vi "Plot Closed.vi"(8 "error in (no error)":errorcluster, 10 "Closed plot":refnum<class "Message Enqueuer.lvclass">, 11 "Measure Controller in":refnum<class "Measure Controller.lvclass">) -> (0 "error out":errorcluster, 3 "Measure Controller out":refnum<class "Measure Controller.lvclass">)   [LabVIEW 2015, in "Measure Controller.lvclass"]
uses:
  Measure Controller.lvclass
  <vilib>/ActorFramework/Message Enqueuer/Message Enqueuer.lvclass
  Measure Controller.lvclass/Measure Controller.ctl
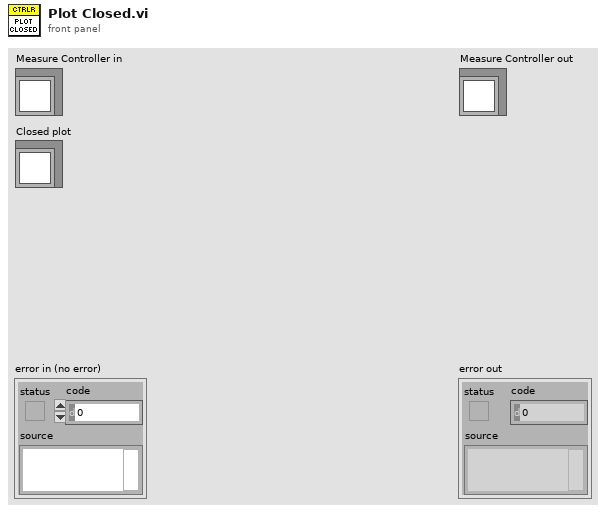
[diagram p1: front panel]
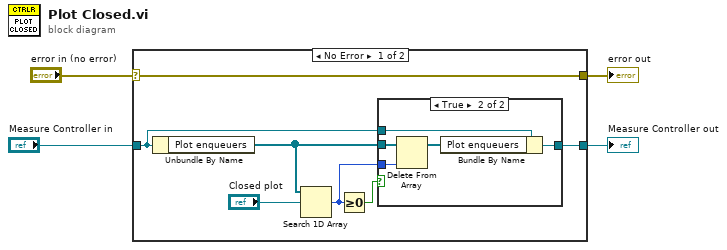
[diagram p0: block diagram]
diagram:
  n1 = case shown="No Error" "error in (no error)" {
    selector: "error in (no error)" -> [w11 w19]
    tunnel: [w11 w19] -> w3
    tunnel: [w5 w18] -> w1
    tunnel: "Measure Controller in" -> [w6 w18]
    frame No Error {
      n2 = Unbundle By Name(w6) -> ("Plot enqueuers"=w9:refnum<class "Message Enqueuer.lvclass">[])
      n3 = Search 1D Array(1D array=w9, element="Closed plot") -> (index of element=w8:i32)  [unwired: 1 in]
      n4 = Greater Or Equal To 0?(x=w8) -> (x >= 0?=w7:bool)
      n5 = case shown="True" w7 {
        tunnel: w9 -> [_ w17]
        tunnel: w8 -> [_ w16]
        tunnel: w6 -> [w12 w15]
        tunnel: [w12 w13] -> w5
        frame False {
        }
        frame True {
          n6 = Delete From Array(array=w17, index=w16) -> (array with subset deleted=w14:refnum<class "Message Enqueuer.lvclass">[])  [unwired: 1 in, 1 out]
          n7 = Bundle By Name(cluster=w15, "Plot enqueuers"=w14) -> (w13:refnum<class "Measure Controller.lvclass">)
        }
      }
    }
    frame Error {
    }
  }
  "error out" <- w3
  "Measure Controller out" <- w1
